vi "JSON text to Variant (Void).vi"(8 "error in (no error)":errorcluster, 9 "Data Type":variant, 10 "Offset":i32, 11 "JSON":string) -> (0 "error out":errorcluster, 1 "Variant out":variant)   [LabVIEW 2021, in "jsontext.facade.lvlib"]
doc: "Convert JSON to the Data Type entered, which may be a cluster or array."
uses:
  jsontext.facade.lvlib
  jsontext/LVClass Serializer/JSONtext LVClass Serializer.lvclass
  jsontext/JSONtext.lvlib
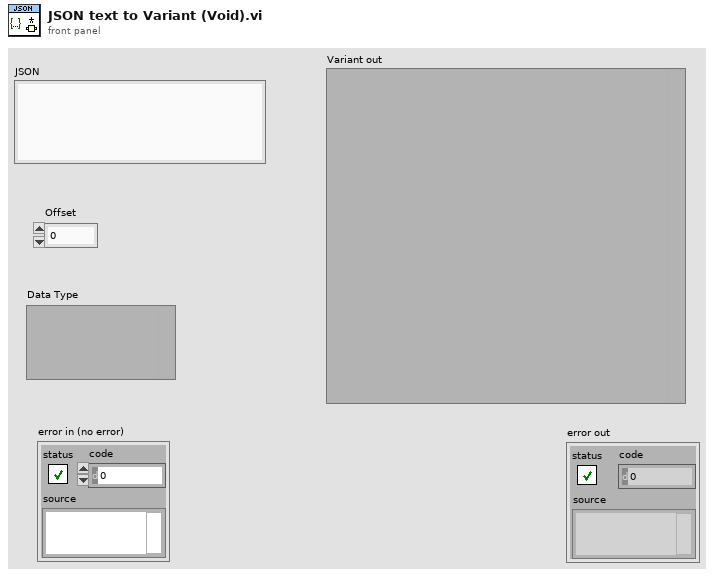
[diagram p1: front panel]
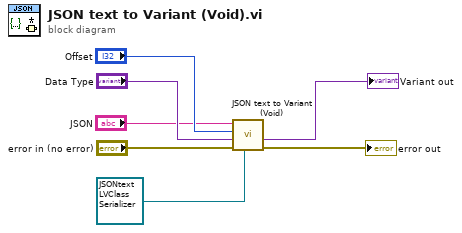
[diagram p0: block diagram]
diagram:
  n1 = call "JSON text to Variant (Void).vi"("LVClass Serializer"=refnum<class "JSONtext LVClass Serializer.lvclass"> refnum, "error in (no error)"="error in (no error)", "Data Type"="Data Type", "Offset"="Offset", "JSON"="JSON") -> ("error out"=→"error out":errorcluster, "Variant out"=→"Variant out":variant)  [unwired: 5 in]
